vi "Array of String_Write Index Set.vi"(9 "Values":cluster{"String Array":string[]}[](array[cluster]), 11 "Indices":i32[](array[numeric])) -> ()   [LabVIEW 2010, in "Current Value Table.lvlib"]
doc: "This VI writes a set of data as defined by the GetIndices function. This VI can provide an order of magnitude increase in performance over a normal index write for sufficiently large data sets."
uses:
  Current Value Table.lvlib
  Type Defs/Memory Commands.ctl
  Array of String_Memory Block.vi
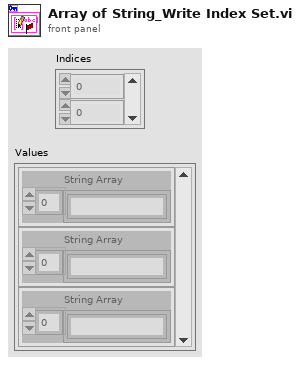
[diagram p1: front panel]
types:
  T1 = typedef "Current Value Table.lvlib/Memory Commands.ctl" = enum16{"Init", "Add Data", "Read", "Read Group", "Read All", "Write", "Write Group", "Get Size"}
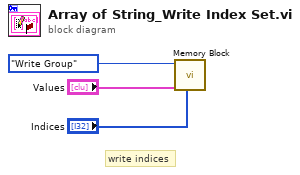
[diagram p0: block diagram]
diagram:
  # "write indices"
  n1 = call-poly "Memory Block.vi"("Group Indices"="Indices", "Data In"="Values", "Method"=Memory_Commands."Write Group") -> ()  [unwired: 6 in, 3 out]
